vi "Client Generator Error Strings Global.vi"() -> ()   [LabVIEW 2021, in "NI Measurement V2 Client Generator Runtime.lvlib"]
uses:
  NI Measurement V2 Client Generator Runtime.lvlib
panel:
  out "5104":string="The measurement plug-in client name '%s' is either already in use or contains invalid characters such as spaces or: \\ / : * ? \" < > |"
  out "5103":string="The provided project path is invalid."
  out "5102":string="The Measurement Plug-In Client generator requires\nInstrumentStudio Professional version 2024 Q4 or higher."
  out "5101":string="Measurements with no configuration or results are not supported by the tool."
  out "5100":string="Internal error. No case found for the control name '%s'."
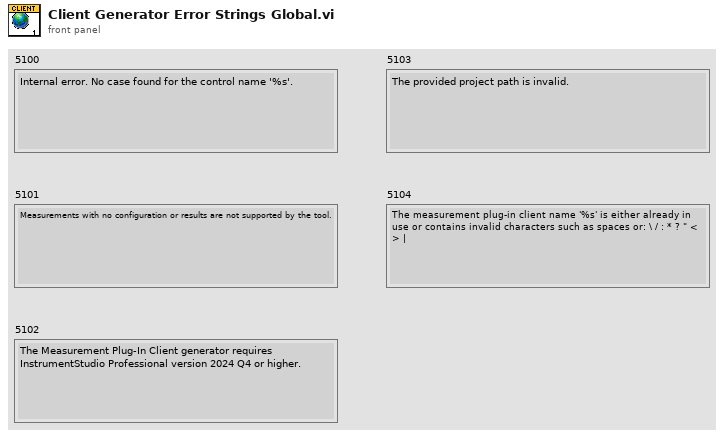
[diagram p1: front panel]
diagram:
